vi "Contour_Setting_UI.vi"(6 "Analysis_Setting In":T1={"PreProcess"=enum."*Algorithm*", "Parameter"=""}, 8 "error in (no error)":errorcluster, 11 "Vision_Image":T3(plugin-control)) -> (0 "error out":errorcluster, 1 "Cancel?":bool, 3 "Analysis_Setting Out":T1={"PreProcess"=enum."*Algorithm*", "Parameter"=""})   [LabVIEW 2019]
uses:
  Controls/_UI Command Cluster/Contour_UICommand.ctl
  <vilib>/Utility/miscctls.llb/LVPointTypeDef.ctl
  <vilib>/vision/Contour.llb/IMAQ Contour Curve Extraction.ctl
  <vilib>/vision/Contour.llb/IMAQ Connect Range Setting.ctl
  Controls/Contour/Analysis_Contour_Parameter.ctl
  Controls/Analysis_Type.ctl
  Controls/Analysis_Setting.ctl
  Controls/V_Analysis_Type.ctl
  Ctrl/VisionProcessName.ctl
panel:
  out "Length":dbl
  in  "ReadImage":bool
  in  "Contour Selection":T4(ring)
  in  "Curve Extraction":T5={"Extraction Mode"=0, "Edge Threshold"=75, "Edge Filter Size"=1, "Min Length"=25, "Search Step Size"=15, "Max Endpoint Gap"=10, "Subpixel"=TRUE} {"Edge Filter Size" items=["Fine", "Normal", "Contour Tracing"]; "Extraction Mode" items=["Normal", "Uniform Regions"]}
  in  "Search Direction":T6(ring)
  in  "Cancel":bool
  in  "OK":bool
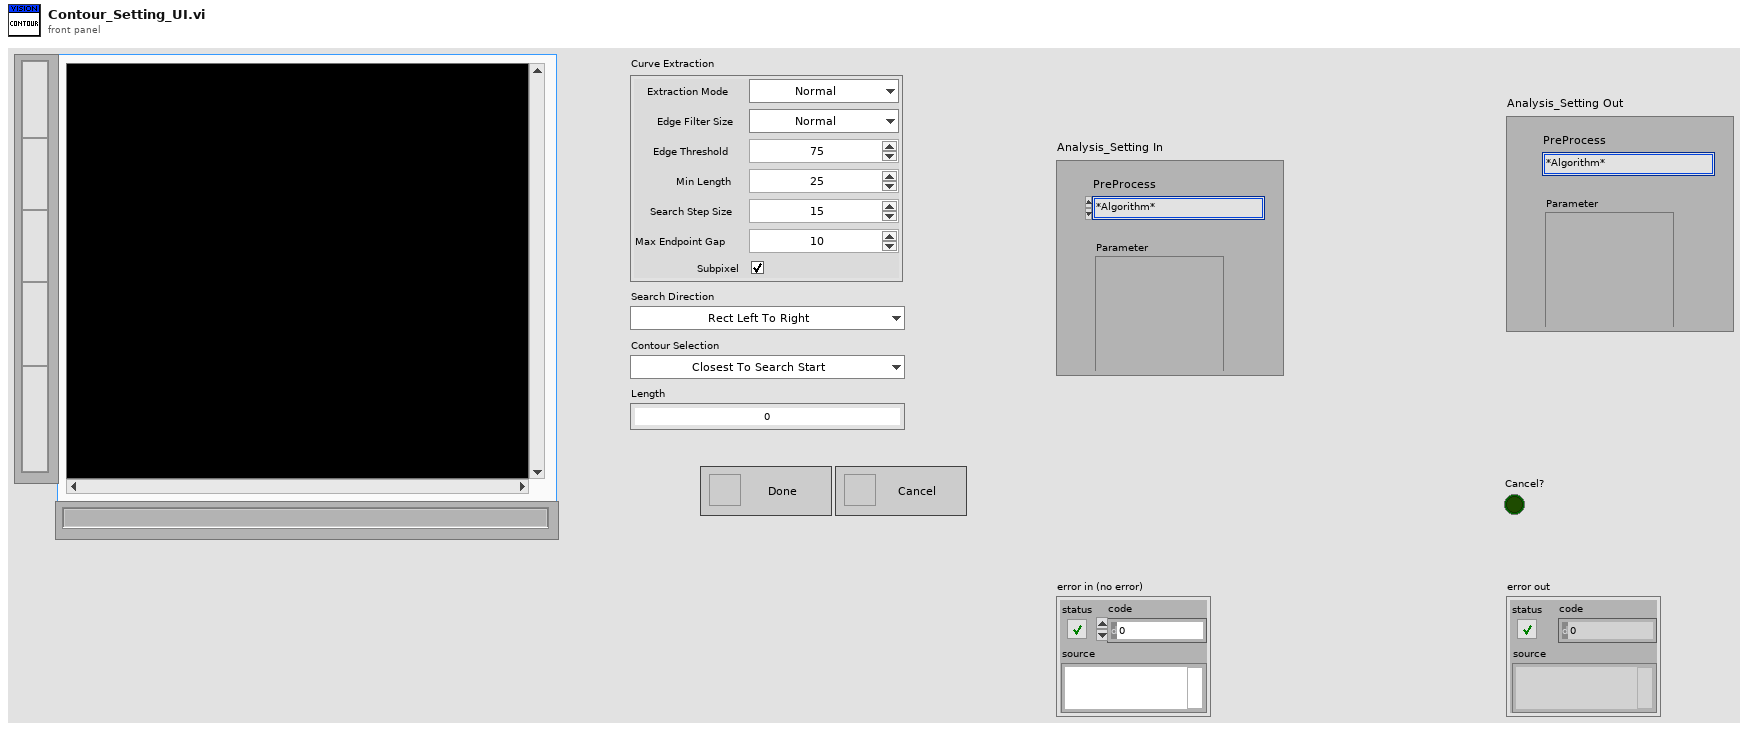
[diagram p1: front panel]
types:
  T1 = typedef "Analysis_Setting.ctl" = cluster{"PreProcess":T2, "Parameter":string}
  T2 = typedef "VisionProcessName.ctl" = enum16{"*CamParameter*", "CamAttributes", "*Preprocess*", "CG_Brightness", "C_Plane Extraction", "C_Threshold", "G_Lookup Table", "G_Threshold", "B_Image Inversion", "*Algorithm*", "CG_Histogram", "C_Color Matching", "C_Color Pattern Matching", "G_PatternMatch", "CG_Find Straight Edge", "CG_Adv. Find Straight Edge", "CG_Find Circular Edge", "G_Max Clamp", "G_Clamp (Rake)", "G_Pattern Matching"}
  T3 = typedef "IMAQ Image.ctl" = refnum<image>
  T4 = enum16{"Closest To Search Start", "Maximum Length", "Strongest Mean Gradient Change"}
  T5 = cluster{"Extraction Mode":u32, "Edge Threshold":i32, "Edge Filter Size":u32, "Min Length":i32, "Search Step Size":i32, "Max Endpoint Gap":i32, "Subpixel":bool}
  T6 = enum16{"Rect Left To Right", "Rect Right To Left", "Rect Top To Bottom", "Rect Bottom To Top", "Annulus Inner To Outer", "Annulus Outer To Inner", "Annulus Start Angle To End Angle", "Annulus End Angle To Start Angle"}
  T7 = typedef "LVPointTypeDef.ctl" = cluster{"Horizontal":i16, "Vertical":i16}
  T8 = typedef "Contour_UICommand.ctl" = cluster{"Message":enum16{"Initialize", "InitializeUI", "CheckDrawTool", "RunAlgorithm", "Done", "Cancel", "Exit"}, "Data":variant}
  T9 = typedef "Analysis_Contour_Parameter.ctl" = cluster{"ROI":cluster{"Global Rectangle":i32[], "Contours":cluster{"ID":enum32{"External", "Internal"}, "Type":u32, "Coordinates":i32[]}[]}, "Search Direction":enum16{"Rect Left To Right", "Rect Right To Left", "Rect Top To Bottom", "Rect Bottom To Top", "Annulus Inner To Outer", "Annulus Outer To Inner", "Annulus Start Angle To End Angle", "Annulus End Angle To Start Angle"}, "Curve Extraction":T10, "Contour Selection":enum16{"Closest To Search Start", "Maximum Length", "Strongest Mean Gradient Change"}, "Curve Connection":T11[]}
  T10 = typedef "IMAQ Contour Curve Extraction.ctl" = cluster{"Extraction Mode":u32, "Edge Threshold":i32, "Edge Filter Size":u32, "Min Length":i32, "Search Step Size":i32, "Max Endpoint Gap":i32, "Subpixel":bool}
  T11 = typedef "IMAQ Connect Range Setting.ctl" = cluster{"Match Constraints":u32, "Min":dbl, "Max":dbl}
  T12 = typedef "Analysis_Setting.ctl" = cluster{"PreProcess":T13, "Parameter":string}
  T13 = typedef "V_Analysis_Type.ctl" = enum16{"None", "C_Color Pattern Matching", "G_PatternMatching", "G_ShapeDectect", "G_GeometricMatch", "B_Area Check"}
  T14 = enum16{"Initialize", "InitializeUI", "CheckDrawTool", "RunAlgorithm", "Done", "Cancel", "Exit"}
  T15 = typedef "Image Type" = u32
  T16 = typedef "Analysis_Type.ctl" = u16
  T17 = cluster{"Global Rectangle":i32[], "Contours":cluster{"ID":enum32{"External", "Internal"}, "Type":u32, "Coordinates":i32[]}[]}
  T18 = cluster{"Global Rectangle":i32[], "Contours":cluster{"Contour Type":u32, "ROI Type":u32, "Points":i32[]}[]}
  T19 = typedef "Analysis_Contour_Result.ctl" = cluster{"Points (pixel)":cluster{"X":dbl, "Y":dbl}[], "Points (real)":cluster{"X":dbl, "Y":dbl}[], "Length (pixel)":dbl, "Length (real)":dbl}
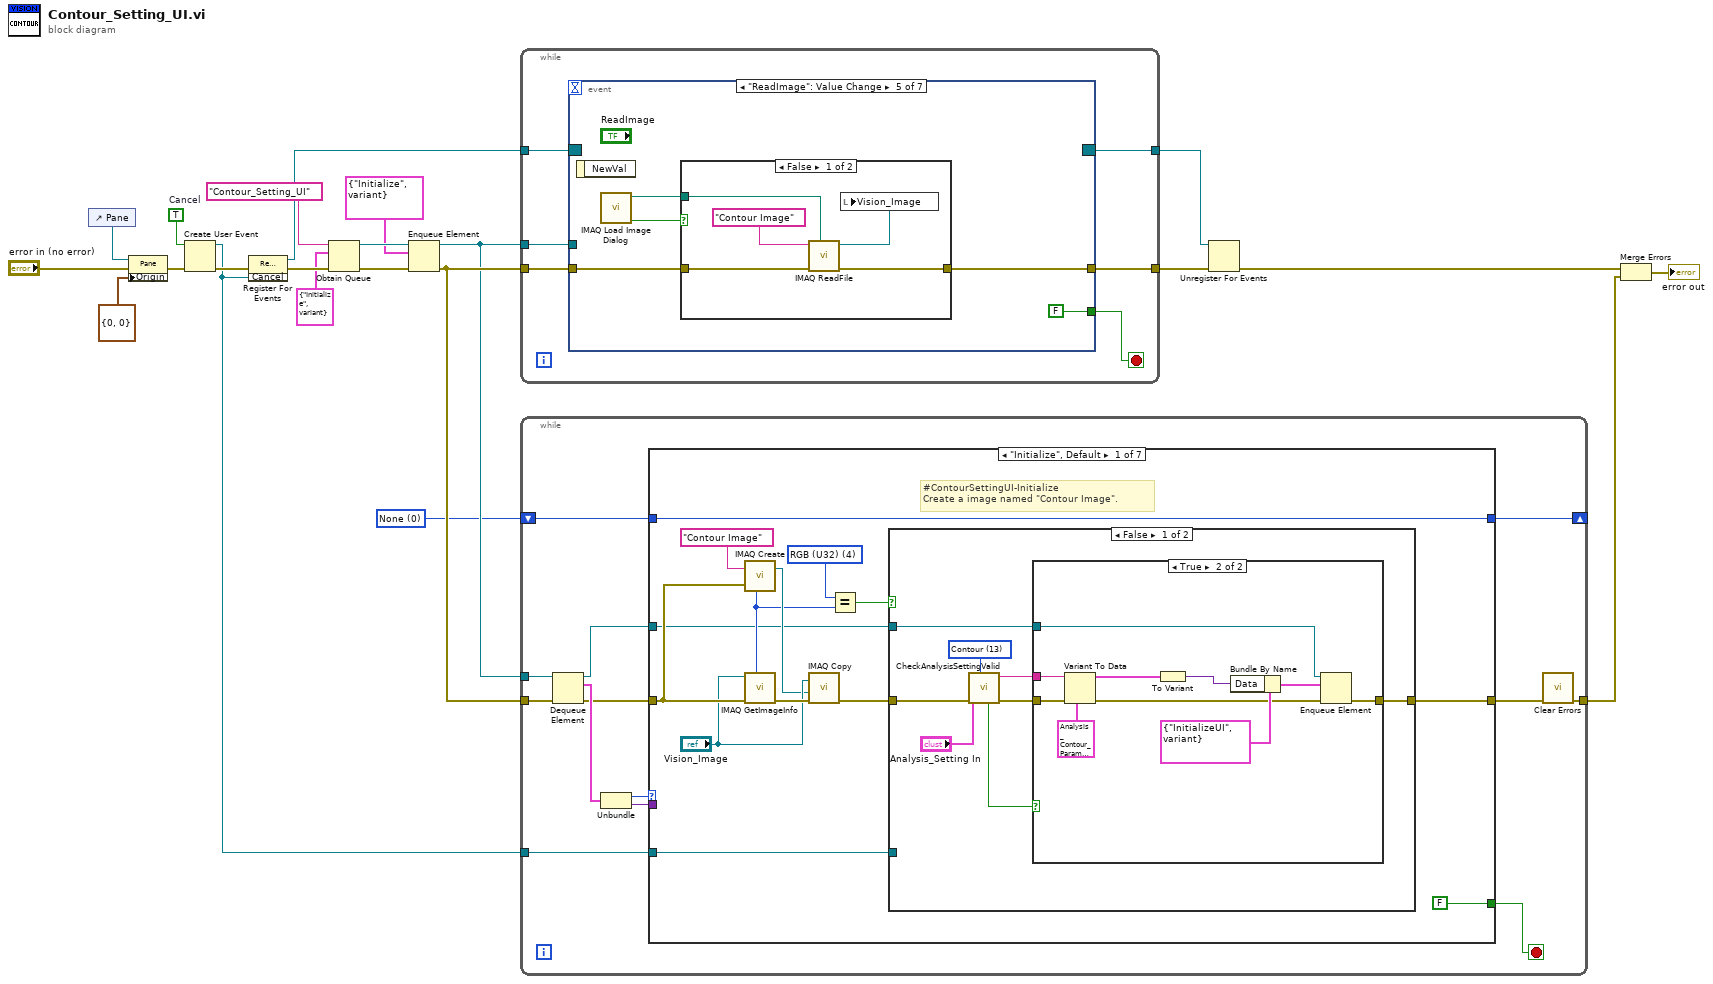
[diagram p0: block diagram]
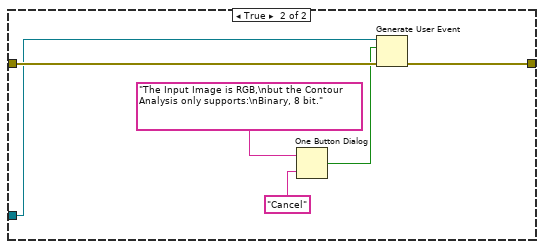
[diagram p3: hidden frame]
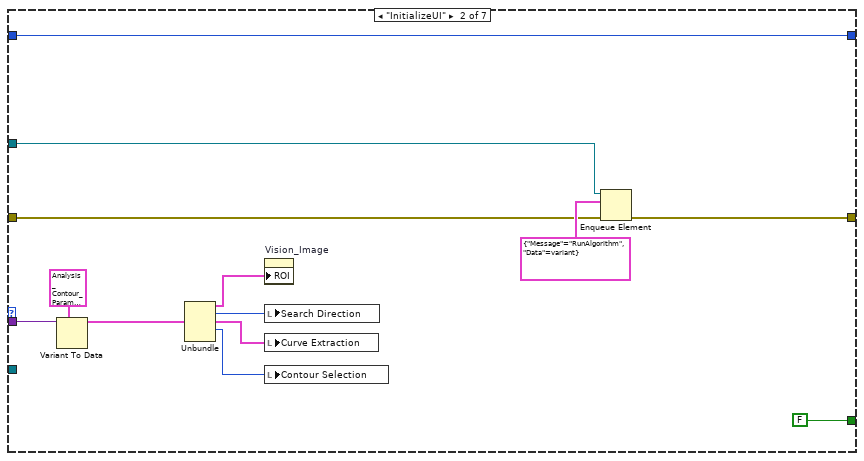
[diagram p4: hidden frame]
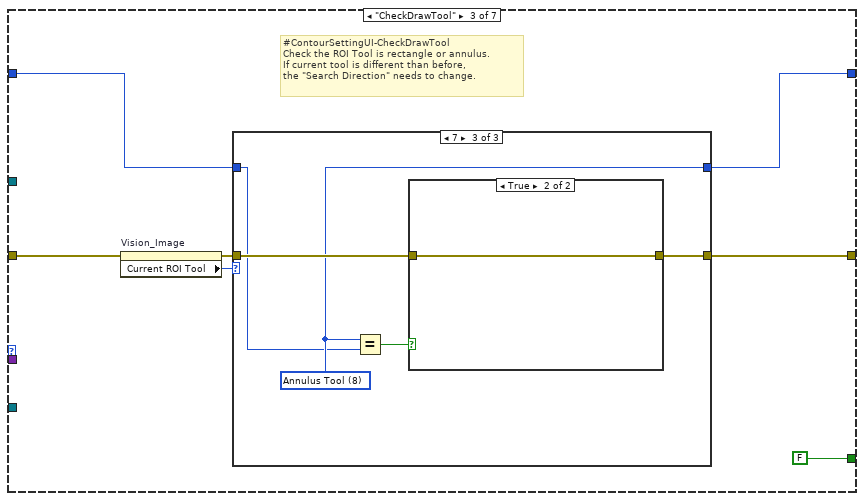
[diagram p5: hidden frame]
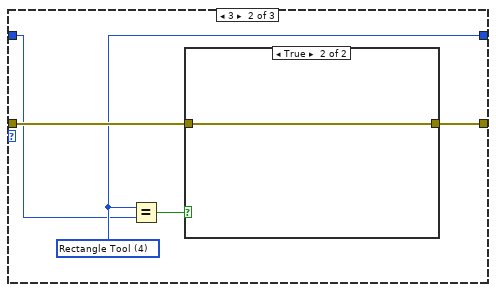
[diagram p7: hidden frame]
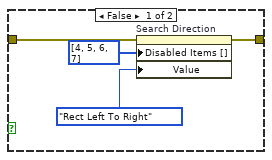
[diagram p8: hidden frame]
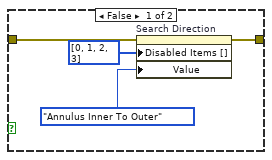
[diagram p9: hidden frame]
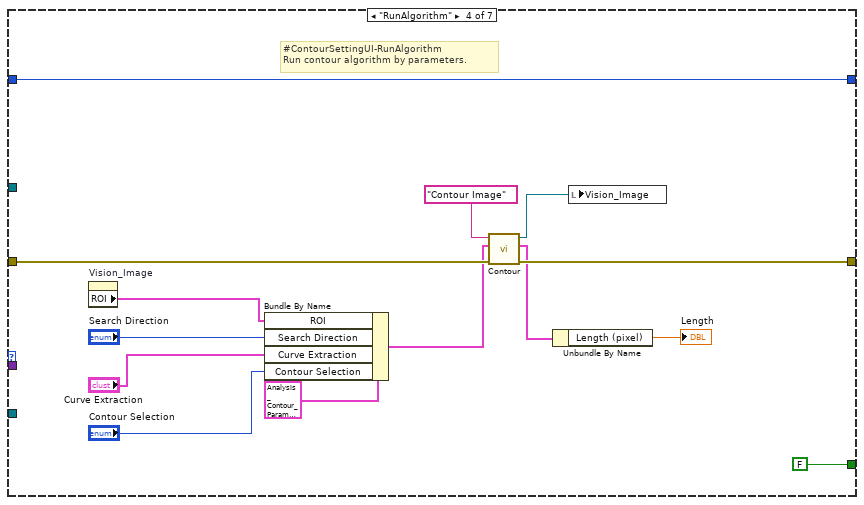
[diagram p10: hidden frame]
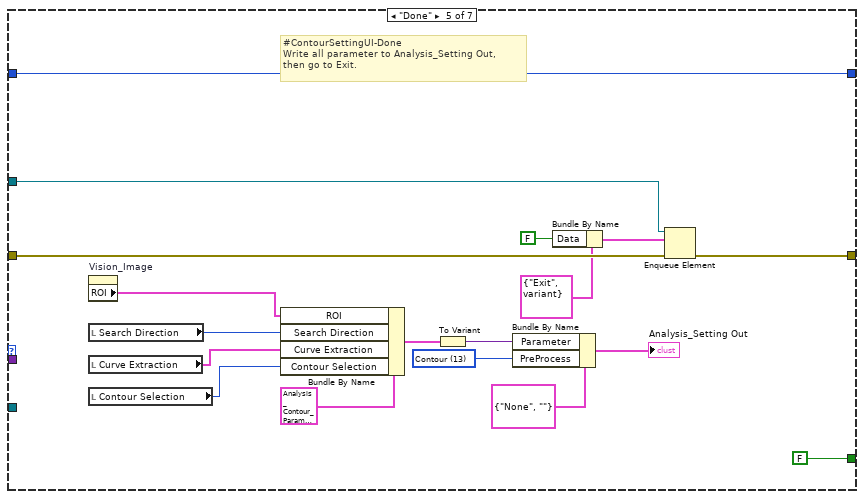
[diagram p11: hidden frame]
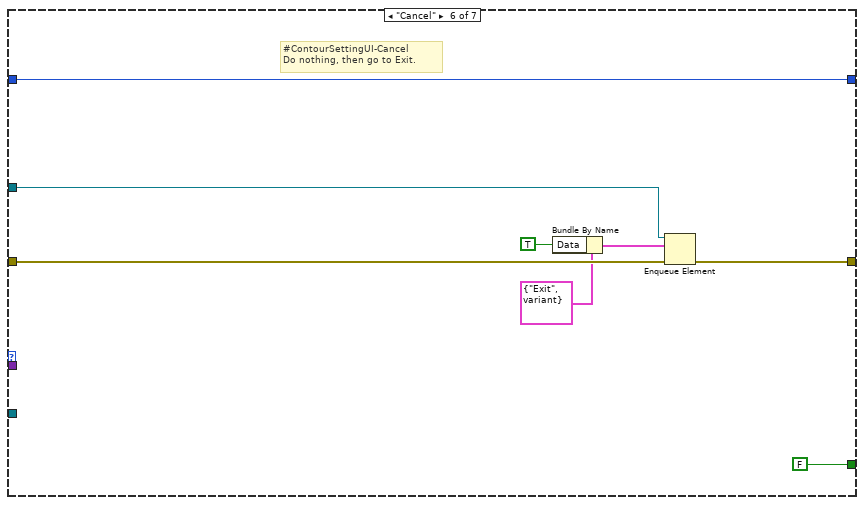
[diagram p12: hidden frame]
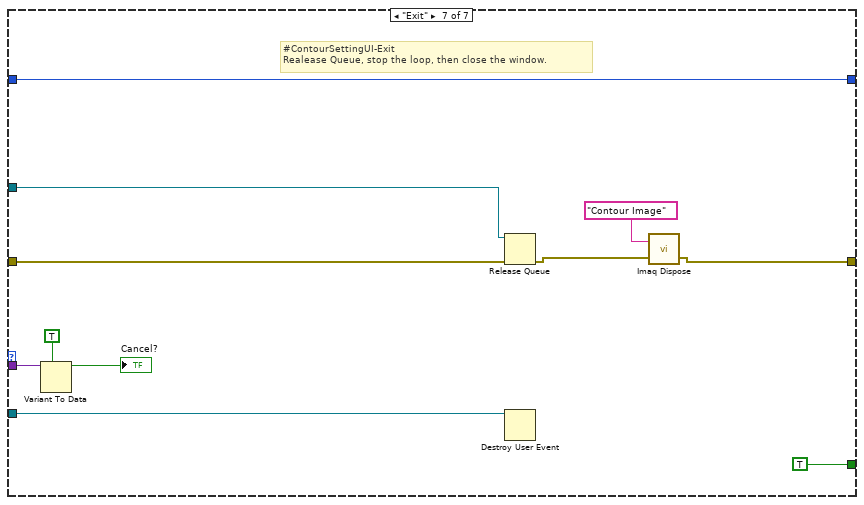
[diagram p13: hidden frame]
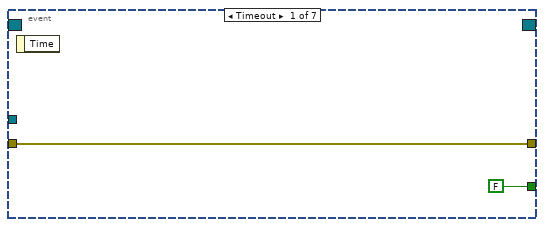
[diagram p14: hidden frame]
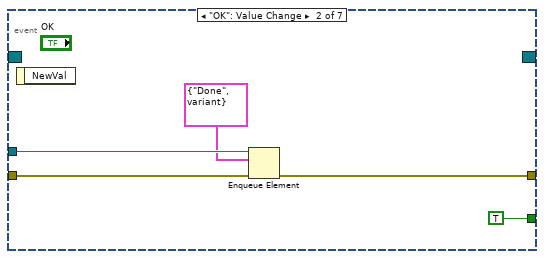
[diagram p15: hidden frame]
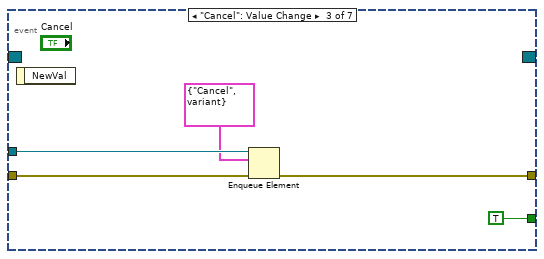
[diagram p16: hidden frame]
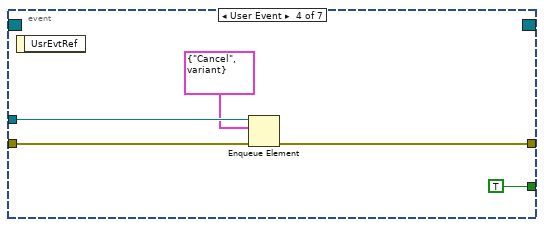
[diagram p17: hidden frame]
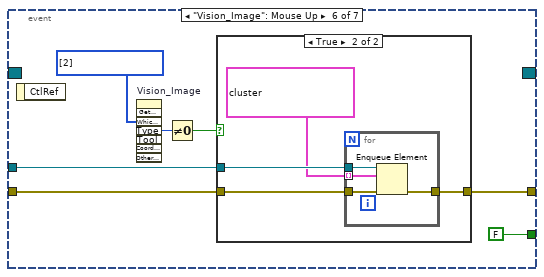
[diagram p19: hidden frame]
diagram:
  w6 = 0 items=["None", "Selection Tool", "Point Tool", "Line Tool", "Rectangle Tool", "Oval Tool", "Polygon Tool", "ClosedFreehandTool", "Annulus Tool", "Rotated Rectangle Tool", "Zoom Tool", "Pan Tool", "Polyline Tool", "Freehand Tool"] ("Tool")
  w16 = TRUE  # Cancel
  n1 = control-ref of="Pane"() -> (w9:refnum<vi>)
  n2 = property class="Pane"(reference=w9, error in="error in (no error)", "Origin"=T7 {"Horizontal"=0, "Vertical"=0}) -> (error out=w8:errorcluster)  [unwired: 1 out]
  n3 = Create User Event(user event datatype=w16, error in=w8) -> (user event=w10:refnum<user-event>, error out=w17:errorcluster)
  n4 = register-events(error in=w17, w10) -> (reference out=w15:refnum<event-registration>, error out=w18:errorcluster)  [unwired: 1 in]
  n5 = Obtain Queue(name (unnamed)="Contour_Setting_UI", element data type=T8 {"Message"=enum."Initialize", "Data"=variant} ("_UICommand"), error in (no error)=w18) -> (queue out=w21:refnum<queue>, error out=w22:errorcluster)  [unwired: 2 in, 1 out]
  n6 = Enqueue Element(queue=w21, element=T8 {"Message"=enum."Initialize", "Data"=variant} ("_UICommand"), error in (no error)=w22) -> (queue out=w19:refnum<queue>, error out=w20:errorcluster)  [unwired: 1 in, 1 out]
  n7 = while {
    tunnel: w19 -> [w28]
    tunnel: w20 -> [w27]
    tunnel: w15 -> [w26]
    tunnel: [w25] -> w14
    tunnel: [w24] -> w13
    stop <- w23 stop-if-true
    n8 = event shown="[4] \"ReadImage\": Value Change" {
      selector: w26 -> [_ _ _ _ _ _ _]
      dyn-events: [_ _ _ _ _ _ _] -> w25
      timeout: _ -> [_ _ _ _ _ _ _]
      tunnel: w28 -> [_ w33 w38 w45 _ w61 w76]
      tunnel: w27 -> [w30 w34 w40 w44 w50 w60 w75]
      tunnel: [w30 w35 w39 w43 w49 w59 w74] -> w24
      tunnel: [FALSE TRUE TRUE TRUE FALSE FALSE FALSE] -> w23
      event Timeout {
        n9 = event-data() -> ()  [unwired: 1 in, 1 out]
      }
      event "OK": Value Change {
        n10 = event-data() -> ()  [unwired: 1 in, 1 out]
        n11 = Enqueue Element(queue=w33, element=T8 {"Message"=enum."Done", "Data"=variant} ("_UICommand"), error in (no error)=w34) -> (error out=w35:errorcluster)  [unwired: 1 in, 2 out]
      }
      event "Cancel": Value Change {
        n12 = event-data() -> ()  [unwired: 1 in, 1 out]
        n13 = Enqueue Element(queue=w38, element=T8 {"Message"=enum."Cancel", "Data"=variant} ("_UICommand"), error in (no error)=w40) -> (error out=w39:errorcluster)  [unwired: 1 in, 2 out]
      }
      event User Event {
        n14 = event-data() -> ()  [unwired: 1 in, 1 out]
        n15 = Enqueue Element(queue=w45, element=T8 {"Message"=enum."Cancel", "Data"=variant} ("_UICommand"), error in (no error)=w44) -> (error out=w43:errorcluster)  [unwired: 1 in, 2 out]
      }
      event "ReadImage": Value Change {
        n16 = event-data() -> ()  [unwired: 1 in, 1 out]
        n17 = call "IMAQ Load Image Dialog"() -> ("Cancelled?"=w47:bool, "Path"=w46:path)  [unwired: 9 in, 1 out]
        n18 = case shown="False" w47 {
          tunnel: w50 -> [w55 w56]
          tunnel: [w54 w56] -> w49
          tunnel: w46 -> [w52 _]
          frame False {
            n19 = call "IMAQ ReadFile"("File Path"=w52, "error in (no error)"=w55, "Image"="Contour Image" ("Image Name")) -> ("error out"=w54:errorcluster, "Image Out"=w51:T3)  [unwired: 4 in, 3 out]
            n20 = local write "Vision_Image"(w51) -> ()
          }
          frame True {
          }
        }
      }
      event "Vision_Image": Mouse Up {
        w57 = i32[] [2] items=["No Event"=0, "Click Event"=1, "Draw Event"=2, "Size Event"=4, "Scroll Event"=5, "Double Click Event"=8] ("Which Events")
        n21 = event-data() -> ()  [unwired: 1 in, 1 out]
        n22 = invoke on="Vision_Image" class="ImageControl" method="Get Last Event"("Which Events"=w57) -> ("Type"=w63:i32)  [unwired: 7 in, 7 out]
        n23 = Not Equal To 0?(x=w63) -> (x != 0?=w62:bool)
        n24 = case shown="True" w62 {
          tunnel: w61 -> [_ w68]
          tunnel: w60 -> [w64 w67]
          tunnel: [w64 w66] -> w59
          frame False {
          }
          frame True {
            n25 = for {
              tunnel: w68 -> [w72]
              tunnel: w67 -> [w71]
              tunnel: [w70] -> w66
              tunnel: T8[] [{"Message"=enum."CheckDrawTool", "Data"=variant}, {"Message"=enum."RunAlgorithm", "Data"=variant}] -> [w69] mode=indexing
              n26 = Enqueue Element(queue=w72, element=w69, error in (no error)=w71) -> (error out=w70:errorcluster)  [unwired: 1 in, 2 out]
            }
          }
        }
      }
      event "Curve Extraction", "Search Direction", "Contour Selection": Value Change {
        n27 = event-data() -> ()  [unwired: 1 in, 1 out]
        n28 = Enqueue Element(queue=w76, element=T8 {"Message"=enum."RunAlgorithm", "Data"=variant} ("_UICommand"), error in (no error)=w75) -> (error out=w74:errorcluster)  [unwired: 1 in, 2 out]
      }
    }
  }
  n29 = while {
    tunnel: w20 -> [w90]
    tunnel: w19 -> [w89]
    tunnel: w10 -> [w83]
    shift-right: [w80] -> _
    shift-left: w6 -> [w81]
    tunnel: [w79] -> w2
    stop <- w82 stop-if-true
    n30 = Dequeue Element(queue=w89, error in (no error)=w90) -> (queue out=w87:refnum<queue>, element=w88:T8, error out=w85:errorcluster)  [unwired: 1 in, 1 out]
    n31 = Unbundle(w88) -> ("Message"=w86:T14, "Data"=w84:variant)
    n32 = case shown="\"Initialize\", Default" w86 {
      tunnel: w87 -> [w91 w130 _ _ w199 w207 w215]
      tunnel: w85 -> [w101 w132 w148 w184 w202 w210 w222]
      tunnel: w84 -> [_ w140 _ _ _ _ w214]
      tunnel: [FALSE FALSE FALSE FALSE FALSE FALSE TRUE] -> w82
      tunnel: w83 -> [w92 _ _ _ _ _ w220]
      tunnel: [w94 w131 w144 w176 w201 w209 w217] -> w78
      tunnel: w81 -> [w102 w142 w145 w174 w200 w208 w216]
      tunnel: [w102 w142 w143 w174 w200 w208 w216] -> w80
      frame "Initialize", Default {
        w95 = T15 4 items=["Grayscale (U8)", "Grayscale (I16)", "Grayscale (SGL)", "Complex (CSG)", "RGB (U32)", "HSL (U32)", "RGB (U64)", "Grayscale (U16)"] ("x")
        # "#ContourSettingUI-Initialize\nCreate a image named \"Contour Image\"."
        n33 = call "IMAQ GetImageInfo"("error in (no error)"=w101, "Image"="Vision_Image") -> ("error out"=w100:errorcluster, "Image Type"=w96:T15)  [unwired: 2 in, 6 out]
        n34 = call "IMAQ Create"("Image Name"="Contour Image", "Image Type"=w96, "error in (no error)"=w101) -> ("New Image"=w97:T3)  [unwired: 2 in, 1 out]
        n35 = call "IMAQ Copy"("error in (no error)"=w100, "Image Dst"=w97, "Image Src"="Vision_Image") -> ("error out"=w99:errorcluster)  [unwired: 3 in, 1 out]
        n36 = Equal?(x=w95, y=w96) -> (x = y?=w93:bool)
        n37 = case shown="False" w93 {
          tunnel: w99 -> [w111 w129]
          tunnel: [w108 w124] -> w94
          tunnel: w92 -> [_ w128]
          tunnel: w91 -> [w106 _]
          frame False {
            w110 = T16 13 items=["None", "PatternMatch", "Edge Detection", "Barcode 1D", "Barcode 2D", "Clamp", "Clamp MAX", "Particle", "Histogram", "Straight Edge", "Circle", "Shape Detect", "OCR", "Contour", "ColorMatch"] ("Analysis_Type")
            n38 = call "CheckAnalysisSettingValid.vi"("Analysis_Type"=w110, "error in (no error)"=w111, "ParameterIn"="Analysis_Setting In") -> ("error out"=w109:errorcluster, "ParameterOut"=w105:string, "Valid"=w107:bool)  [unwired: 6 in]
            n39 = case shown="True" w107 {
              tunnel: w109 -> [w113 w123]
              tunnel: [w113 w122] -> w108
              tunnel: w106 -> [_ w119]
              tunnel: w105 -> [_ w120]
              frame False {
              }
              frame True {
                n40 = Variant To Data(error in=w123, type=T9 {"ROI"={"Global Rectangle"=[], "Contours"=[]}, "Search Direction"=enum."Rect Left To Right", "Curve Extraction"={"Extraction Mode"=0, "Edge Threshold"=75, "Edge Filter Size"=1, "Min Length"=25, "Search Step Size"=15, "Max Endpoint Gap"=10, "Subpixel"=TRUE}, "Contour Selection"=enum."Closest To Search Start", "Curve Connection"=[]} ("ContourParameter"), Variant=w120) -> (data=w117:T9, error out=w114:errorcluster)
                n41 = To Variant(anything=w117) -> (Variant=w116:variant)
                n42 = Bundle By Name(cluster=T8 {"Message"=enum."InitializeUI", "Data"=variant} ("_UICommand"), "Data"=w116) -> (w115:T8)
                n43 = Enqueue Element(queue=w119, element=w115, error in (no error)=w114) -> (error out=w122:errorcluster)  [unwired: 1 in, 2 out]
              }
            }
          }
          frame True {
            n44 = One Button Dialog(message="The Input Image is RGB,\nbut the Contour Analysis only supports:\nBinary, 8 bit.", button name ("OK")="Cancel") -> (true=w125:bool)
            n45 = Generate User Event(user event=w128, event data cluster=w125, error in=w129) -> (error out=w124:errorcluster)  [unwired: 1 in, 1 out]
          }
        }
      }
      frame "InitializeUI" {
        n46 = Variant To Data(type=T9 {"ROI"={"Global Rectangle"=[], "Contours"=[]}, "Search Direction"=enum."Rect Left To Right", "Curve Extraction"={"Extraction Mode"=0, "Edge Threshold"=75, "Edge Filter Size"=1, "Min Length"=25, "Search Step Size"=15, "Max Endpoint Gap"=10, "Subpixel"=TRUE}, "Contour Selection"=enum."Closest To Search Start", "Curve Connection"=[]} ("ContourParameter"), Variant=w140) -> (data=w137:T9)  [unwired: 1 in, 1 out]
        n47 = Unbundle(w137) -> ("ROI"=w134:T17, "Search Direction"=w136:T6, "Curve Extraction"=w135:T10, "Contour Selection"=w138:T4)  [unwired: 1 out]
        n48 = property on="Vision_Image" class="ImageControl"("ROI"=w134) -> ()  [unwired: 2 in, 2 out]
        n49 = local write "Search Direction"(w136) -> ()
        n50 = local write "Curve Extraction"(w135) -> ()
        n51 = local write "Contour Selection"(w138) -> ()
        n52 = Enqueue Element(queue=w130, element=T8 {"Message"=enum."RunAlgorithm", "Data"=variant} ("_UICommand"), error in (no error)=w132) -> (error out=w131:errorcluster)  [unwired: 1 in, 2 out]
      }
      frame "CheckDrawTool" {
        # "#ContourSettingUI-CheckDrawTool\nCheck the ROI Tool is rectangle or annulus.\nIf current tool is different than before,\nthe \"Search Direction\" needs to change."
        n53 = property on="Vision_Image" class="ImageControl"(error in=w148) -> (error out=w146:errorcluster, "Current ROI Tool"=w147:u32)  [unwired: 1 in, 1 out]
        n54 = case shown="7" w147 {
          tunnel: w146 -> [w151 w155 w165]
          tunnel: w145 -> [w150 w152 w162]
          tunnel: [w151 w154 w164] -> w144
          tunnel: [w150 w153 w163] -> w143
          frame Default {
          }
          frame 3 {
            w153 = 4 items=["None", "Selection Tool", "Point Tool", "Line Tool", "Rectangle Tool", "Oval Tool", "Polygon Tool", "ClosedFreehandTool", "Annulus Tool", "Rotated Rectangle Tool", "Zoom Tool", "Pan Tool", "Polyline Tool", "Freehand Tool"] ("Tool")
            n55 = Equal?(x=w153, y=w152) -> (x = y?=w156:bool)
            n56 = case shown="True" w156 {
              tunnel: w155 -> [w159 w161]
              tunnel: [w158 w161] -> w154
              frame False {
                n57 = property on="Search Direction" class="Enum (strict)"(error in=w159, "Disabled Items []"=i32[] [4, 5, 6, 7], "Value"=T6."Rect Left To Right" ("Search Direction")) -> (error out=w158:errorcluster)  [unwired: 1 in, 1 out]
              }
              frame True {
              }
            }
          }
          frame 7 {
            w163 = 8 items=["None", "Selection Tool", "Point Tool", "Line Tool", "Rectangle Tool", "Oval Tool", "Polygon Tool", "ClosedFreehandTool", "Annulus Tool", "Rotated Rectangle Tool", "Zoom Tool", "Pan Tool", "Polyline Tool", "Freehand Tool"] ("Tool")
            n58 = Equal?(x=w163, y=w162) -> (x = y?=w166:bool)
            n59 = case shown="True" w166 {
              tunnel: w165 -> [w169 w171]
              tunnel: [w168 w171] -> w164
              frame False {
                n60 = property on="Search Direction" class="Enum (strict)"(error in=w169, "Disabled Items []"=i32[] [0, 1, 2, 3], "Value"=T6."Annulus Inner To Outer" ("Search Direction")) -> (error out=w168:errorcluster)  [unwired: 1 in, 1 out]
              }
              frame True {
              }
            }
          }
        }
      }
      frame "RunAlgorithm" {
        # "#ContourSettingUI-RunAlgorithm\nRun contour algorithm by parameters."
        n61 = property on="Vision_Image" class="ImageControl"() -> ("ROI"=w173:T18)  [unwired: 2 in, 2 out]
        n62 = Bundle By Name(cluster=T9 {"ROI"={"Global Rectangle"=[], "Contours"=[]}, "Search Direction"=enum."Rect Left To Right", "Curve Extraction"={"Extraction Mode"=0, "Edge Threshold"=75, "Edge Filter Size"=1, "Min Length"=25, "Search Step Size"=15, "Max Endpoint Gap"=10, "Subpixel"=TRUE}, "Contour Selection"=enum."Closest To Search Start", "Curve Connection"=[]} ("ContourParameter"), "ROI"=w173, "Search Direction"="Search Direction", "Curve Extraction"="Curve Extraction", "Contour Selection"="Contour Selection") -> (w177:T9)
        n63 = call "Contour.vi"("error in (no error)"=w184, "ContourParameter"=w177, "Image In"="Contour Image" ("Image Name")) -> ("error out"=w176:errorcluster, "ContourResult"=w175:T19, "Image Out"=w182:T3)  [unwired: 6 in]
        n64 = Unbundle By Name(w175) -> ("Length (pixel)"=→"Length":dbl)
        n65 = local write "Vision_Image"(w182) -> ()
      }
      frame "Done" {
        w187 = T16 13 items=["None", "PatternMatch", "Edge Detection", "Barcode 1D", "Barcode 2D", "Clamp", "Clamp MAX", "Particle", "Histogram", "Straight Edge", "Circle", "Shape Detect", "OCR", "Contour", "ColorMatch"] ("Analysis_Type")
        # "#ContourSettingUI-Done\nWrite all parameter to Analysis_Setting Out,\nthen go to Exit."
        n66 = property on="Vision_Image" class="ImageControl"() -> ("ROI"=w194:T18)  [unwired: 2 in, 2 out]
        n67 = local read "Search Direction"() -> (w193:T6)
        n68 = local read "Curve Extraction"() -> (w192:T5)
        n69 = local read "Contour Selection"() -> (w191:T4)
        n70 = Bundle By Name(cluster=T9 {"ROI"={"Global Rectangle"=[], "Contours"=[]}, "Search Direction"=enum."Rect Left To Right", "Curve Extraction"={"Extraction Mode"=0, "Edge Threshold"=75, "Edge Filter Size"=1, "Min Length"=25, "Search Step Size"=15, "Max Endpoint Gap"=10, "Subpixel"=TRUE}, "Contour Selection"=enum."Closest To Search Start", "Curve Connection"=[]} ("ContourParameter"), "ROI"=w194, "Search Direction"=w193, "Curve Extraction"=w192, "Contour Selection"=w191) -> (w189:T9)
        n71 = To Variant(anything=w189) -> (Variant=w186:variant)
        n72 = Bundle By Name(cluster=T12 {"PreProcess"=enum."None", "Parameter"=""} ("Analysis_Setting"), "Parameter"=w186, "PreProcess"=w187) -> (→"Analysis_Setting Out":T12)
        n73 = Bundle By Name(cluster=T8 {"Message"=enum."Exit", "Data"=variant} ("_UICommand"), "Data"=FALSE) -> (w196:T8)
        n74 = Enqueue Element(queue=w199, element=w196, error in (no error)=w202) -> (error out=w201:errorcluster)  [unwired: 1 in, 2 out]
      }
      frame "Cancel" {
        # "#ContourSettingUI-Cancel\nDo nothing, then go to Exit."
        n75 = Bundle By Name(cluster=T8 {"Message"=enum."Exit", "Data"=variant} ("_UICommand"), "Data"=TRUE) -> (w205:T8)
        n76 = Enqueue Element(queue=w207, element=w205, error in (no error)=w210) -> (error out=w209:errorcluster)  [unwired: 1 in, 2 out]
      }
      frame "Exit" {
        # "#ContourSettingUI-Exit\nRealease Queue, stop the loop, then close the window."
        n77 = Variant To Data(type=TRUE, Variant=w214) -> (data=→"Cancel?":bool)  [unwired: 1 in, 1 out]
        n78 = Release Queue(queue=w215, error in (no error)=w222) -> (error out=w218:errorcluster)  [unwired: 1 in, 2 out]
        n79 = Destroy User Event(user event=w220) -> ()  [unwired: 1 in, 1 out]
        n80 = call "Imaq Dispose"("Image"="Contour Image" ("Image Name"), "error in (no error)"=w218) -> ("error out"=w217:errorcluster)  [unwired: 4 in]
      }
    }
    n81 = call <vilib>:"Clear Errors.vi"("error in (no error)"=w78) -> ("error out"=w79:errorcluster)  [unwired: 5 in, 1 out]
  }
  n82 = Unregister For Events(event registration refnum=w14, error in=w13) -> (error out=w3:errorcluster)
  n83 = Merge Errors(w3, w2) -> (→"error out":errorcluster)
